vi "Auton Commands.vi"(7 "Roll":dbl, 8 "Turn Angle":dbl, 9 "Distance":dbl=120.0, 10 "Task":u16(ring) items=["Forward", "Backward", "Turn", "Shoot", "Turn Angle", "Roll G", "Roll L"]) -> ()   [LabVIEW 2015]
uses:
  <vilib>/Rock Robotics/Network Tables/NT Read Number.vi
  <vilib>/Rock Robotics/WPI/Utilities/WPI_GetSetVariantRefNum.vi
  <vilib>/addons/control/pid/pid.llb/PID (DBL).vi
  <vilib>/Rock Robotics/Network Tables/NT Write Number.vi
  Robot Global Data.vi
  <vilib>/addons/control/pid/NI_PID_pid.lvlib
  navX Library v2/navX Library v2.lvlib
panel:
  out "Yaw":dbl(graph)
  out "E1 Rate":dbl
  out "E2 Rate":dbl
  in  "Yaw Gains":T1={"proportional gain (Kc)"=0.2, "integral time (Ti, min)"=0.0, "derivative time (Td, min)"=0.0} {"derivative time (Td, min)" format="%.3f"; "integral time (Ti, min)" format="%.3f"; "proportional gain (Kc)" format="%.3f"}
  in  "Speed Gains":T1={"proportional gain (Kc)"=0.65, "integral time (Ti, min)"=0.001, "derivative time (Td, min)"=0.001} {"derivative time (Td, min)" format="%.3f"; "integral time (Ti, min)" format="%.3f"; "proportional gain (Kc)" format="%.3f"}
  in  "Single Turn Gains":T1={"proportional gain (Kc)"=0.12, "integral time (Ti, min)"=0.0, "derivative time (Td, min)"=0.0} {"derivative time (Td, min)" format="%.3f"; "integral time (Ti, min)" format="%.3f"; "proportional gain (Kc)" format="%.3f"}
  out "Right Motor Speed":dbl(graph)
  out "Left Motor Speed":dbl(graph)
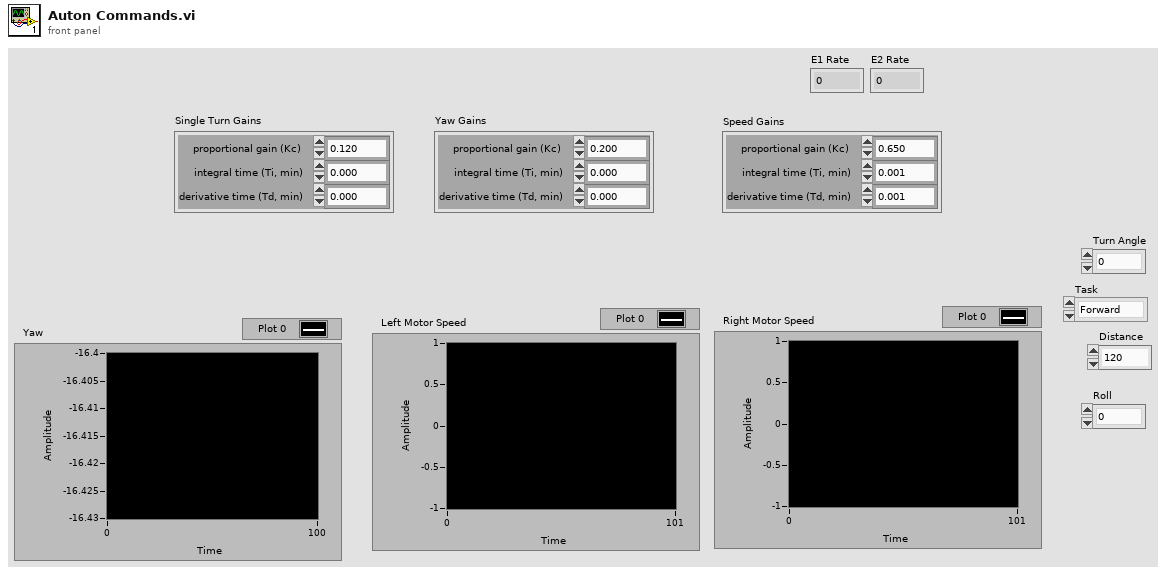
[diagram p1: front panel]
types:
  T1 = cluster{"proportional gain (Kc)":dbl, "integral time (Ti, min)":dbl, "derivative time (Td, min)":dbl}
  T2 = typedef "navX Library v2.lvlib/Z900_navX_DeviceTypeDef.ctl" = cluster{"Interface":cluster{"Protocol":T3, "Update Rate (4Hz-60Hz)":u8, "navX Open TypeDef":variant}, "Notify Packet":refnum<notifier>, "Loop VI Refnum":refnum<vi>, "Ready to Close Occurrence Refnum":refnum<k4>}
  T3 = typedef "navX Library v2.lvlib/Z900_navX_ProtocolTypeDef.ctl" = enum16{"SERIAL", "I2C", "SPI"}
  T4 = typedef "WPI_EncoderDevRef.ctl" = cluster{"DevStatus":errorcluster, "EncoderIndex":T5, "CounterIndex":T6, "DistancePerCount":dbl, "Decoding Type":T7}
  T5 = typedef "FPGA_EncoderIdx.ctl" = enum8{"Enc 0", "Enc 1", "Enc 2", "Enc 3", "Enc 4", "Enc 5", "Enc 6", "Enc 7", "Invalid"}
  T6 = typedef "FPGA_CounterCtrSystemIndex.ctl" = enum8{"Ctr 0", "Ctr 1", "Ctr 2", "Ctr 3", "Ctr 4", "Ctr 5", "Ctr 6", "Ctr 7", "Invalid"}
  T7 = typedef "WPI_EncoderType.ctl" = enum16{"1x", "2x", "4x"}
  T8 = cluster{"Yaw":dbl, "Roll":dbl, "Pitch":dbl, "Heading":dbl, "Fused Heading":dbl}
  T9 = typedef "WPI_RobotDriveDevRef.ctl" = cluster{"DevStatus":errorcluster, "Motors[]":T10[], "Square Inputs":bool, "Max Output":dbl}
  T10 = typedef "WPI_MotorControlDeviceRef.ctl" = cluster{"DeviceStatus":errorcluster, "Type":T11, "PWM":cluster{"PWM Channel":T12, "DeadBand":T13}, "CAN":cluster{"Device Number":u8, "Control Mode":T14, "Semaphore":T15, "Max Vout":dbl, "TalonSRX Control Mode":T16}, "Invert":bool}
  T11 = typedef "WPI_MotorControlType.ctl" = enum16{"PWM", "CAN", "CANTalonSRX"}
  T12 = typedef "FPGA_DIOPWMChannel.ctl" = enum8{"PWM 0", "PWM 1", "PWM 2", "PWM 3", "PWM 4", "PWM 5", "PWM 6", "PWM 7", "PWM 8", "PWM 9", "PWM MXP 0", "PWM MXP 1", "PWM MXP 2", "PWM MXP 3", "PWM MXP 4", "PWM MXP 5", "PWM MXP 6", "PWM MXP 7", "PWM MXP 8", "PWM MXP 9", "Invalid"}
  T13 = typedef "WPI_PWMDeadband.ctl" = cluster{"Name":string, "maxPositivePwm":i32, "minPositivePwm":i32, "centerPwm":i32, "maxNegativePwm":i32, "minNegativePwm":i32, "angularRange":u16}
  T14 = typedef "WPI_CANJaguar_ControlMode.ctl" = enum8{"Percent VBus", "Current", "Speed", "Position", "Voltage"}
  T15 = typedef "Semaphore RefNum" = refnum<k1>
  T16 = typedef "WPI_CANTalonSRX_APIControlMode.ctl" = enum8{"Percent VBus", "Speed", "Position", "Slave", "Unchanged / Invalid", "Voltage Compensation", "Current", "Motion Profile"}
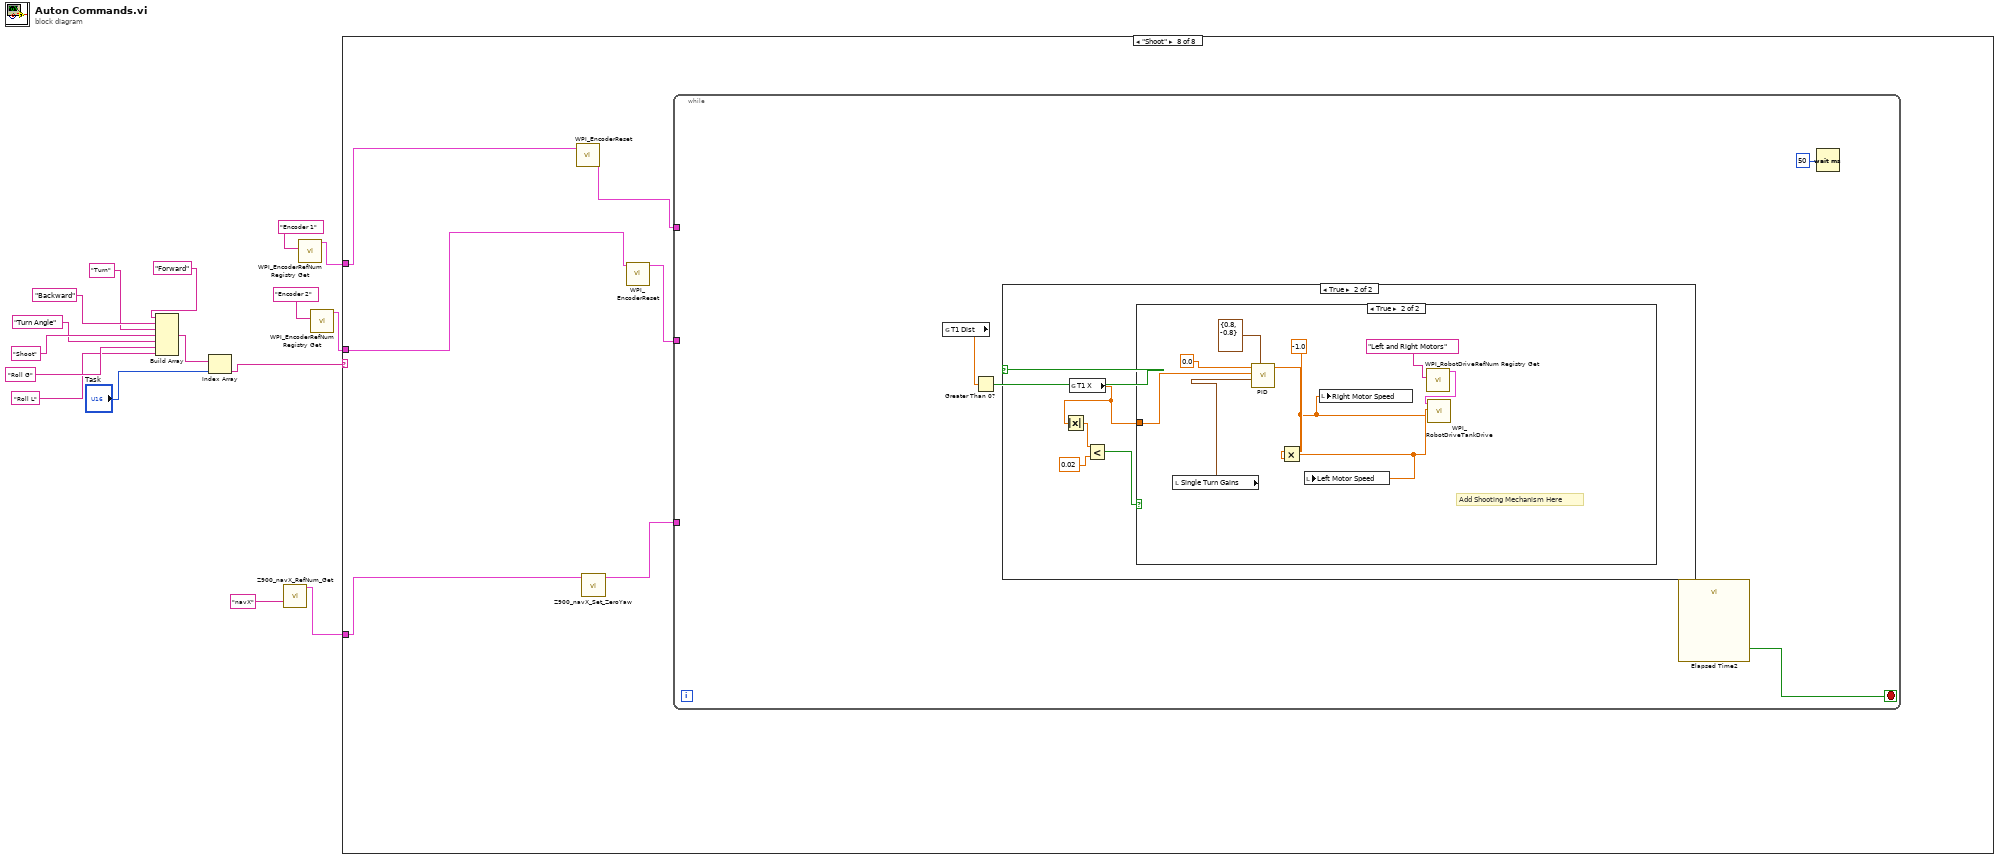
[diagram p0: block diagram]
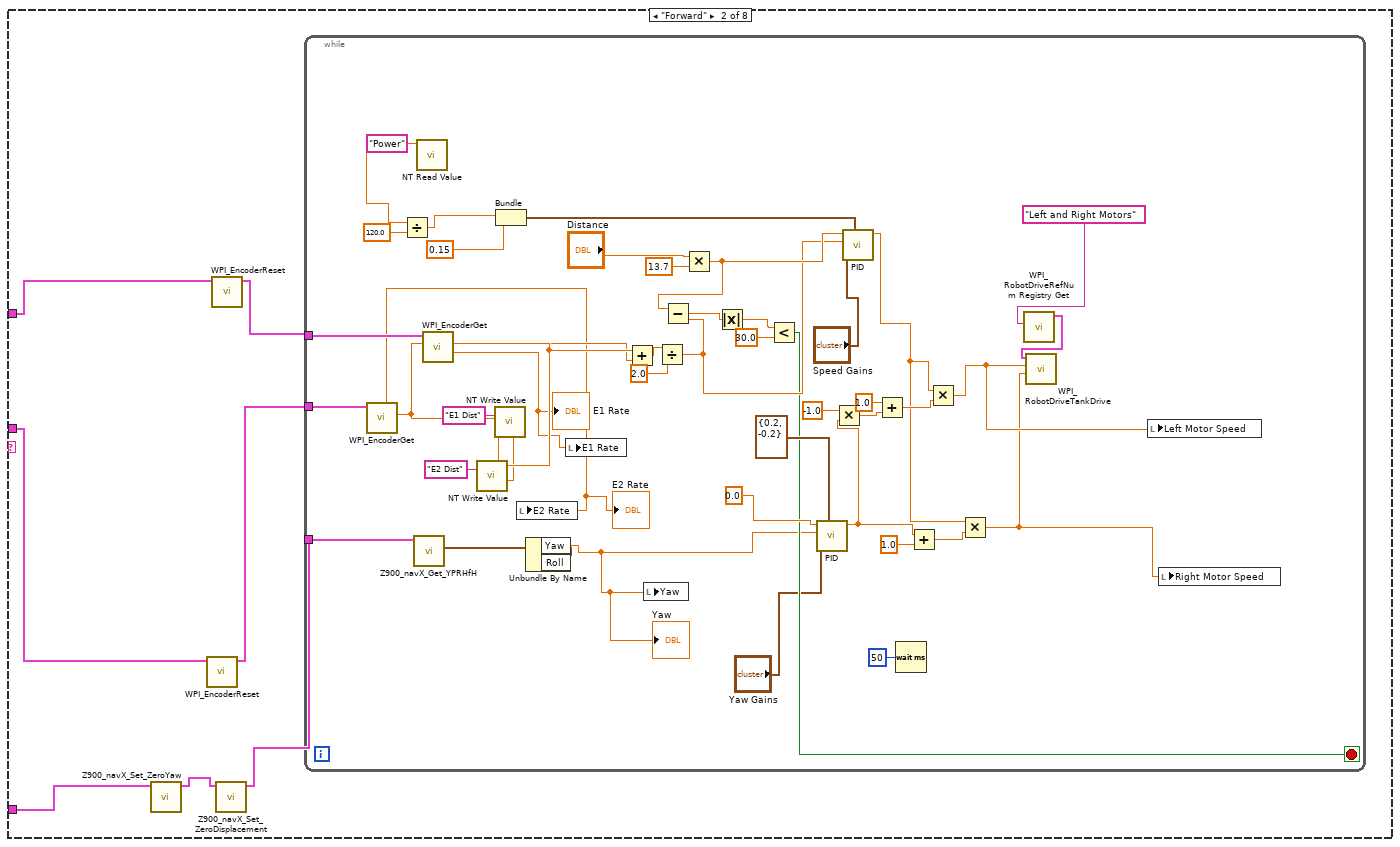
[diagram p3: hidden frame]
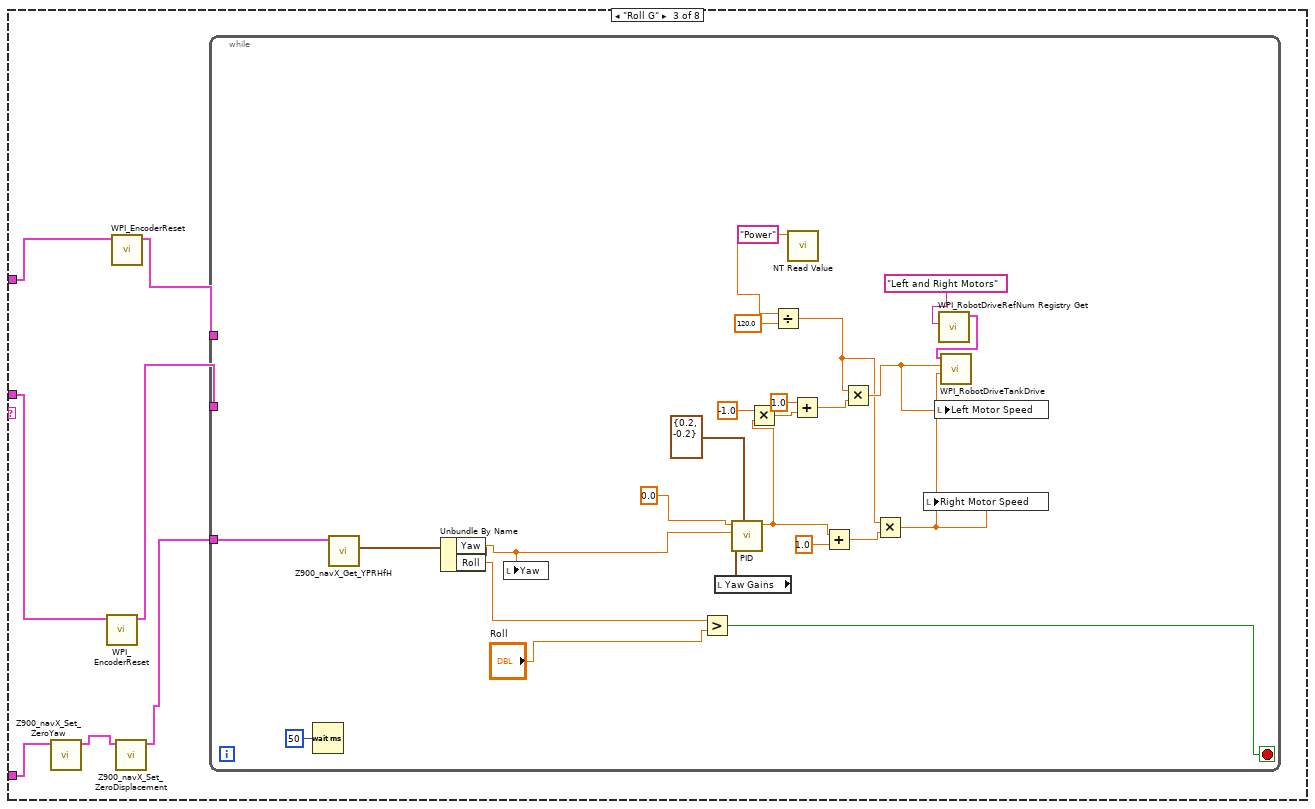
[diagram p4: hidden frame]
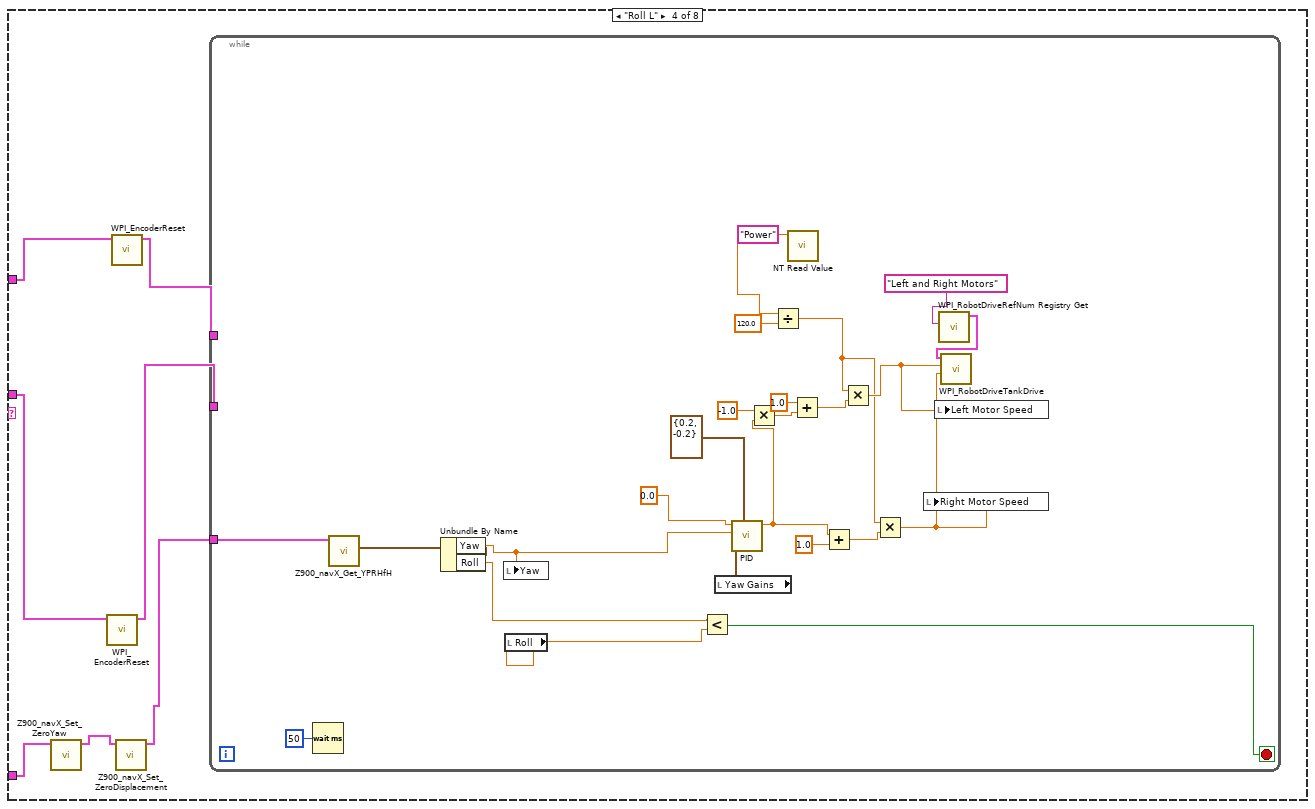
[diagram p5: hidden frame]
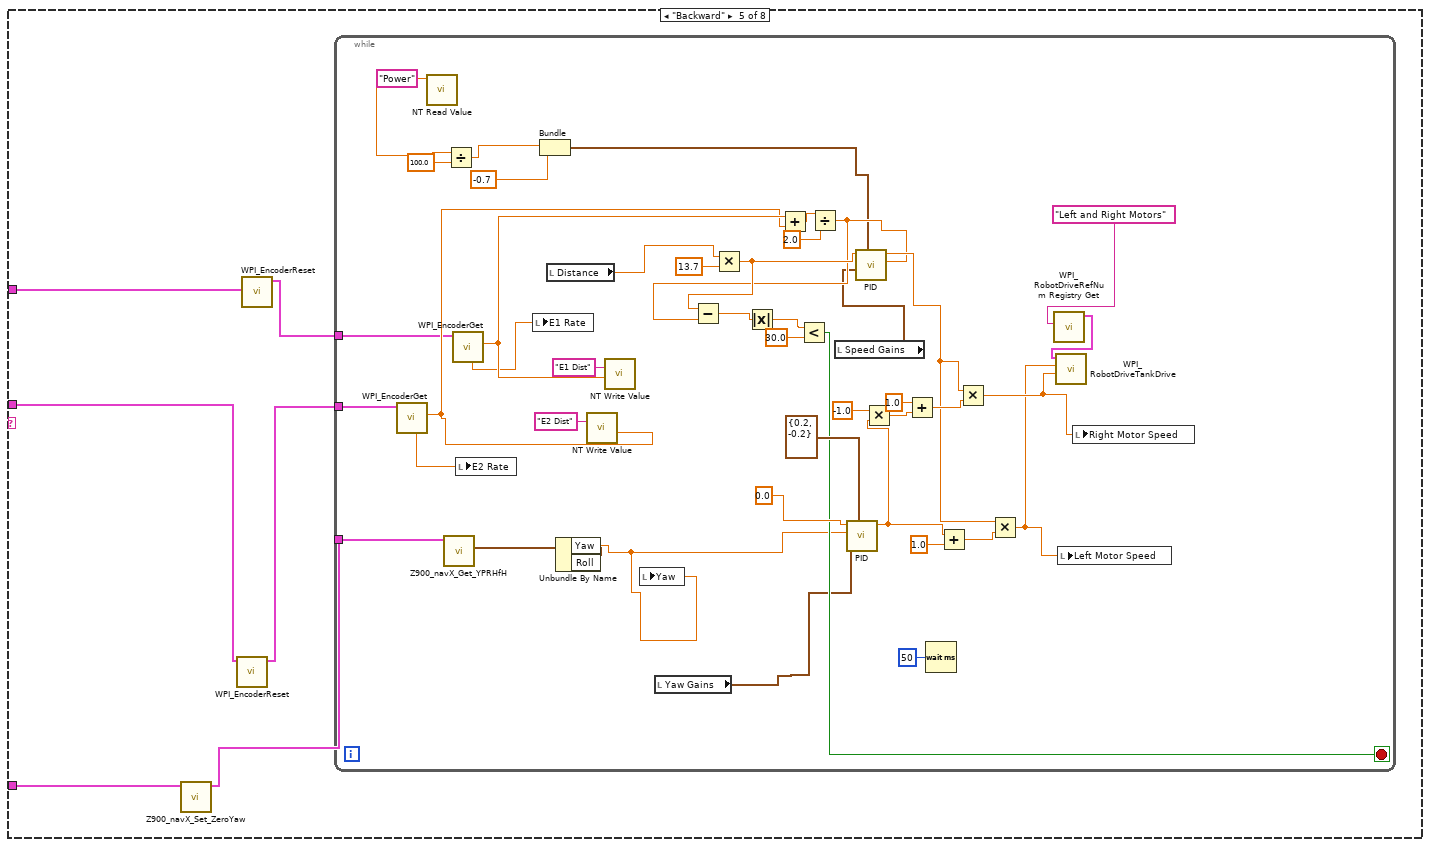
[diagram p6: hidden frame]
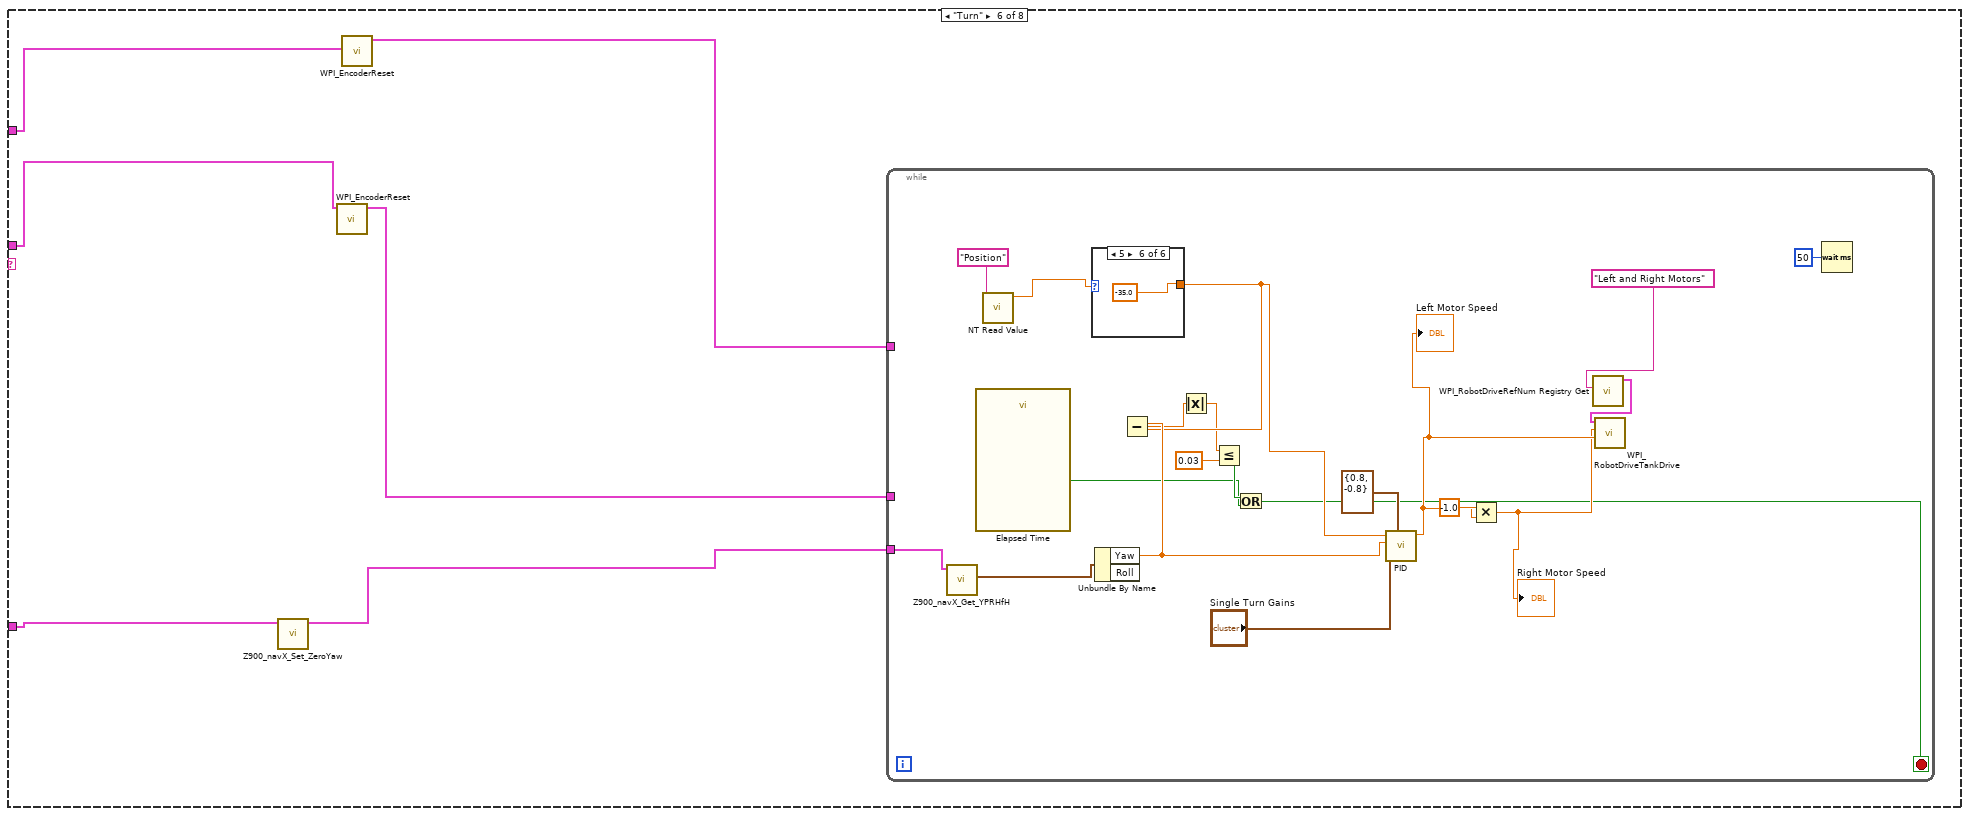
[diagram p7: hidden frame]
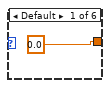
[diagram p8: hidden frame]
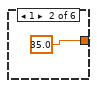
[diagram p9: hidden frame]
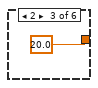
[diagram p10: hidden frame]
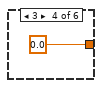
[diagram p11: hidden frame]
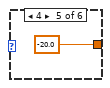
[diagram p12: hidden frame]
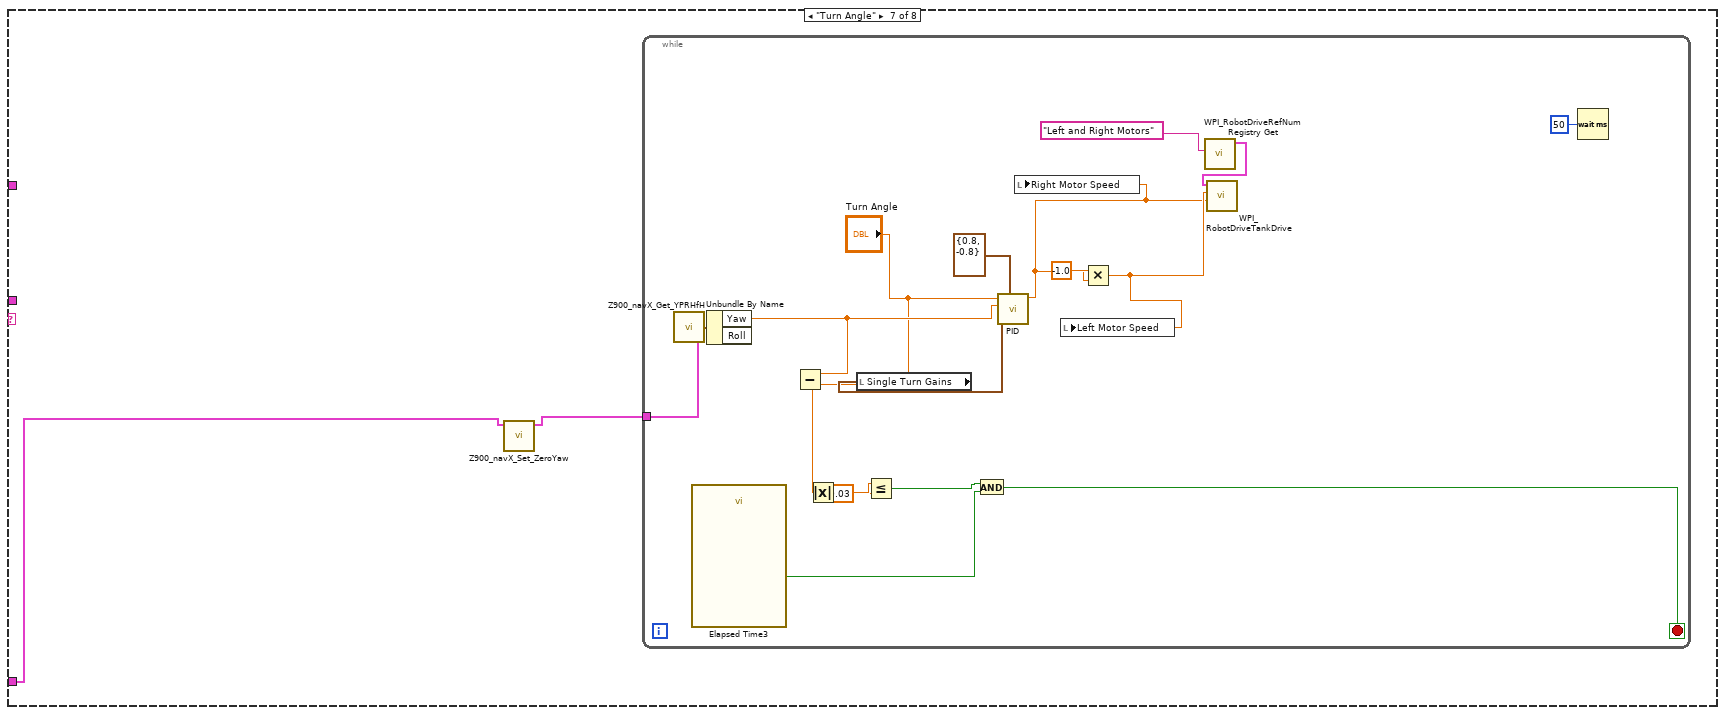
[diagram p13: hidden frame]
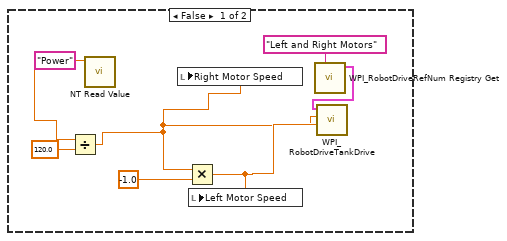
[diagram p14: hidden frame]
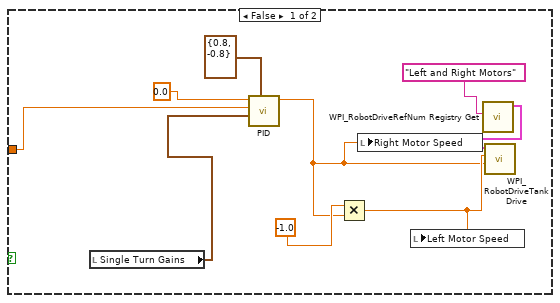
[diagram p15: hidden frame]
diagram:
  n1 = Build Array("Forward", "Backward", "Turn", "Shoot", "Turn Angle" ("element"), "Roll G" ("element"), "Roll L" ("element")) -> (w10:string[])
  n2 = Index Array(array=w10, index="Task") -> (element=w8:string)
  n3 = call "Z900_navX_RefNum_Get.vi"("refnum name"="navX") -> ("navX Device"=w11:T2)  [unwired: 9 in, 1 out]
  n4 = call <vilib>:"WPI_EncoderRefNum Registry Get.vi"("refnum name"="Encoder 1") -> ("EncoderDevRef"=w15:T4)  [unwired: 9 in, 1 out]
  n5 = call <vilib>:"WPI_EncoderRefNum Registry Get.vi"("refnum name"="Encoder 2") -> ("EncoderDevRef"=w13:T4)  [unwired: 9 in, 1 out]
  n6 = case shown="\"Shoot\"" w8 {
    tunnel: w15 -> [_ w21 w73 w105 w134 w184 _ w237]
    tunnel: w13 -> [_ w20 w70 w102 w133 w183 _ w236]
    tunnel: w11 -> [_ w19 w68 w100 w132 w182 w214 w235]
    frame Default {
    }
    frame "Forward" {
      n7 = call "Z900_navX_Set_ZeroYaw.vi"("navX Device"=w19) -> ("navX Device"=w18:T2)  [unwired: 9 in, 1 out]
      n8 = call <vilib>:"WPI_EncoderReset.vi"("EncoderDevRef"=w20) -> ("EncoderDevRef"=w22:T4)  [unwired: 9 in, 1 out]
      n9 = call <vilib>:"WPI_EncoderReset.vi"("EncoderDevRef"=w21) -> ("EncoderDevRef"=w23:T4)  [unwired: 9 in, 1 out]
      n10 = call "Z900_navX_Set_ZeroDisplacement.vi"("navX Device"=w18) -> ("navX Device"=w17:T2)  [unwired: 9 in, 1 out]
      n11 = while {
        tunnel: w23 -> [w34]
        tunnel: w22 -> [w33]
        tunnel: w17 -> [w25]
        stop <- w40 stop-if-true
        n12 = call <vilib>:"WPI_EncoderGet.vi"("EncoderDevRef"=w33) -> ("Distance"=w46:dbl, "Rate"=w32:dbl)  [unwired: 5 in, 4 out]
        "E2 Rate" <- w32
        n13 = call "Z900_navX_Get_YPRHfH.vi"("navX Device"=w25) -> ("YRPHfH"=w62:T8)  [unwired: 7 in, 3 out]
        n14 = call-poly <vilib>:"NT Read Value.vi"("Name"="Power") -> ("Numeric"=w39:dbl)  [unwired: 9 in, 1 out]
        n15 = Divide(x=w39, y=120.0) -> (x/y=w37:dbl)
        n16 = call <vilib>:"WPI_EncoderGet.vi"("EncoderDevRef"=w34) -> ("Distance"=w47:dbl, "Rate"=w31:dbl)  [unwired: 5 in, 4 out]
        "E1 Rate" <- w31
        n17 = call-poly <vilib>:"NT Write Value.vi"("Numeric"=w46, "Name"="E2 Dist") -> ()  [unwired: 9 in, 1 out]
        n18 = call-poly <vilib>:"NT Write Value.vi"("Numeric"=w47, "Name"="E1 Dist") -> ()  [unwired: 9 in, 1 out]
        n19 = Bundle(w37, "output low"=0.15) -> (w35:cluster{dbl, "output low":dbl})  [unwired: 1 in]
        n20 = local write "E2 Rate"(w32) -> ()
        n21 = Unbundle By Name(w62) -> ("Yaw"=w28:dbl)  [unwired: 1 out]
        "Yaw" <- w28
        n22 = local write "E1 Rate"(w31) -> ()
        n23 = Add(x=w47, y=w46) -> (x+y=w61:dbl)
        n24 = local write "Yaw"(w28) -> ()
        n25 = Divide(x=w61, y=2.0) -> (x/y=w44:dbl)
        n26 = Multiply(x="Distance", y=13.7) -> (x*y=w45:dbl)
        n27 = Subtract(x=w45, y=w44) -> (x-y=w43:dbl)
        n28 = Absolute Value(x=w43) -> (abs(x)=w42:dbl)
        n29 = Less?(x=w42, y=30.0) -> (x < y?=w40:bool)
        n30 = call-poly <vilib>:"PID.vi"("output range"=cluster{"output high":dbl, "output low":dbl} {"output high"=0.2, "output low"=-0.2}, "PID gains"="Yaw Gains", "process variable"=w28, "setpoint"=0.0) -> ("output"=w54:dbl)  [unwired: 6 in, 1 out]
        n31 = Multiply(x=-1.0, y=w54) -> (x*y=w55:dbl)
        n32 = call-poly <vilib>:"PID.vi"("output range"=w35, "PID gains"="Speed Gains", "process variable"=w44, "setpoint"=w45) -> ("output"=w51:dbl)  [unwired: 6 in, 1 out]
        n33 = Add(x=1.0, y=w55) -> (x+y=w56:dbl)
        n34 = Wait (ms)(milliseconds to wait=u32 50) -> ()  [unwired: 1 out]
        n35 = Add(x=w54, y=1.0) -> (x+y=w57:dbl)
        n36 = Multiply(x=w51, y=w56) -> (x*y=w49:dbl)
        n37 = Multiply(x=w51, y=w57) -> (x*y=w24:dbl)
        n38 = call <vilib>:"WPI_RobotDriveRefNum Registry Get.vi"("refnum name"="Left and Right Motors") -> ("RobotDriveDevRef"=w64:T9)  [unwired: 9 in, 1 out]
        n39 = call <vilib>:"WPI_RobotDriveTankDrive.vi"("Right axis value"=w24, "Left axis value"=w49, "RobotDriveDevRef"=w64) -> ()  [unwired: 6 in, 3 out]
        n40 = local write "Left Motor Speed"(w49) -> ()
        n41 = local write "Right Motor Speed"(w24) -> ()
      }
    }
    frame "Roll G" {
      n42 = call "Z900_navX_Set_ZeroYaw.vi"("navX Device"=w68) -> ("navX Device"=w74:T2)  [unwired: 9 in, 1 out]
      n43 = call <vilib>:"WPI_EncoderReset.vi"("EncoderDevRef"=w70) -> ("EncoderDevRef"=w71:T4)  [unwired: 9 in, 1 out]
      n44 = call <vilib>:"WPI_EncoderReset.vi"("EncoderDevRef"=w73) -> ("EncoderDevRef"=w72:T4)  [unwired: 9 in, 1 out]
      n45 = call "Z900_navX_Set_ZeroDisplacement.vi"("navX Device"=w74) -> ("navX Device"=w69:T2)  [unwired: 9 in, 1 out]
      n46 = while {
        tunnel: w72 -> [_]
        tunnel: w71 -> [_]
        tunnel: w69 -> [w82]
        stop <- w76 stop-if-true
        n47 = Wait (ms)(milliseconds to wait=u32 50) -> ()  [unwired: 1 out]
        n48 = call "Z900_navX_Get_YPRHfH.vi"("navX Device"=w82) -> ("YRPHfH"=w96:T8)  [unwired: 7 in, 3 out]
        n49 = Unbundle By Name(w96) -> ("Yaw"=w80:dbl, "Roll"=w77:dbl)
        n50 = local write "Yaw"(w80) -> ()
        n51 = Greater?(x=w77, y="Roll") -> (0:w76:bool)
        n52 = local read "Yaw Gains"() -> (w81:T1)
        n53 = call-poly <vilib>:"PID.vi"("output range"=cluster{"output high":dbl, "output low":dbl} {"output high"=0.2, "output low"=-0.2}, "PID gains"=w81, "process variable"=w80, "setpoint"=0.0) -> ("output"=w90:dbl)  [unwired: 6 in, 1 out]
        n54 = Multiply(x=-1.0, y=w90) -> (x*y=w91:dbl)
        n55 = call-poly <vilib>:"NT Read Value.vi"("Name"="Power") -> ("Numeric"=w85:dbl)  [unwired: 9 in, 1 out]
        n56 = Divide(x=w85, y=120.0) -> (x/y=w79:dbl)
        n57 = Add(x=1.0, y=w91) -> (x+y=w92:dbl)
        n58 = Add(x=w90, y=1.0) -> (x+y=w93:dbl)
        n59 = Multiply(x=w79, y=w92) -> (x*y=w87:dbl)
        n60 = Multiply(x=w79, y=w93) -> (x*y=w78:dbl)
        n61 = local write "Right Motor Speed"(w78) -> ()
        n62 = local write "Left Motor Speed"(w87) -> ()
        n63 = call <vilib>:"WPI_RobotDriveRefNum Registry Get.vi"("refnum name"="Left and Right Motors") -> ("RobotDriveDevRef"=w98:T9)  [unwired: 9 in, 1 out]
        n64 = call <vilib>:"WPI_RobotDriveTankDrive.vi"("Right axis value"=w78, "Left axis value"=w87, "RobotDriveDevRef"=w98) -> ()  [unwired: 6 in, 3 out]
      }
    }
    frame "Roll L" {
      n65 = call "Z900_navX_Set_ZeroYaw.vi"("navX Device"=w100) -> ("navX Device"=w106:T2)  [unwired: 9 in, 1 out]
      n66 = call <vilib>:"WPI_EncoderReset.vi"("EncoderDevRef"=w102) -> ("EncoderDevRef"=w103:T4)  [unwired: 9 in, 1 out]
      n67 = call <vilib>:"WPI_EncoderReset.vi"("EncoderDevRef"=w105) -> ("EncoderDevRef"=w104:T4)  [unwired: 9 in, 1 out]
      n68 = call "Z900_navX_Set_ZeroDisplacement.vi"("navX Device"=w106) -> ("navX Device"=w101:T2)  [unwired: 9 in, 1 out]
      n69 = while {
        tunnel: w104 -> [_]
        tunnel: w103 -> [_]
        tunnel: w101 -> [w114]
        stop <- w108 stop-if-true
        n70 = Wait (ms)(milliseconds to wait=u32 50) -> ()  [unwired: 1 out]
        n71 = call "Z900_navX_Get_YPRHfH.vi"("navX Device"=w114) -> ("YRPHfH"=w128:T8)  [unwired: 7 in, 3 out]
        n72 = Unbundle By Name(w128) -> ("Yaw"=w112:dbl, "Roll"=w109:dbl)
        n73 = local write "Yaw"(w112) -> ()
        n74 = local read "Roll"() -> (w107:dbl)
        n75 = Less?(x=w109, y=w107) -> (x < y?=w108:bool)
        n76 = local read "Yaw Gains"() -> (w113:T1)
        n77 = call-poly <vilib>:"PID.vi"("output range"=cluster{"output high":dbl, "output low":dbl} {"output high"=0.2, "output low"=-0.2}, "PID gains"=w113, "process variable"=w112, "setpoint"=0.0) -> ("output"=w122:dbl)  [unwired: 6 in, 1 out]
        n78 = Multiply(x=-1.0, y=w122) -> (x*y=w123:dbl)
        n79 = call-poly <vilib>:"NT Read Value.vi"("Name"="Power") -> ("Numeric"=w117:dbl)  [unwired: 9 in, 1 out]
        n80 = Divide(x=w117, y=120.0) -> (x/y=w111:dbl)
        n81 = Add(x=1.0, y=w123) -> (x+y=w124:dbl)
        n82 = Add(x=w122, y=1.0) -> (x+y=w125:dbl)
        n83 = Multiply(x=w111, y=w124) -> (x*y=w119:dbl)
        n84 = Multiply(x=w111, y=w125) -> (x*y=w110:dbl)
        n85 = local write "Right Motor Speed"(w110) -> ()
        n86 = local write "Left Motor Speed"(w119) -> ()
        n87 = call <vilib>:"WPI_RobotDriveRefNum Registry Get.vi"("refnum name"="Left and Right Motors") -> ("RobotDriveDevRef"=w130:T9)  [unwired: 9 in, 1 out]
        n88 = call <vilib>:"WPI_RobotDriveTankDrive.vi"("Right axis value"=w110, "Left axis value"=w119, "RobotDriveDevRef"=w130) -> ()  [unwired: 6 in, 3 out]
      }
    }
    frame "Backward" {
      n89 = call "Z900_navX_Set_ZeroYaw.vi"("navX Device"=w132) -> ("navX Device"=w135:T2)  [unwired: 9 in, 1 out]
      n90 = call <vilib>:"WPI_EncoderReset.vi"("EncoderDevRef"=w133) -> ("EncoderDevRef"=w136:T4)  [unwired: 9 in, 1 out]
      n91 = call <vilib>:"WPI_EncoderReset.vi"("EncoderDevRef"=w134) -> ("EncoderDevRef"=w137:T4)  [unwired: 9 in, 1 out]
      n92 = while {
        tunnel: w137 -> [w149]
        tunnel: w136 -> [w148]
        tunnel: w135 -> [w147]
        stop <- w155 stop-if-true
        n93 = call <vilib>:"WPI_EncoderGet.vi"("EncoderDevRef"=w148) -> ("Distance"=w161:dbl, "Rate"=w143:dbl)  [unwired: 5 in, 4 out]
        n94 = call-poly <vilib>:"NT Read Value.vi"("Name"="Power") -> ("Numeric"=w154:dbl)  [unwired: 9 in, 1 out]
        n95 = call "Z900_navX_Get_YPRHfH.vi"("navX Device"=w147) -> ("YRPHfH"=w176:T8)  [unwired: 7 in, 3 out]
        n96 = Divide(x=w154, y=100.0) -> (x/y=w152:dbl)
        n97 = call <vilib>:"WPI_EncoderGet.vi"("EncoderDevRef"=w149) -> ("Distance"=w162:dbl, "Rate"=w142:dbl)  [unwired: 5 in, 4 out]
        n98 = local write "E2 Rate"(w143) -> ()
        n99 = local write "E1 Rate"(w142) -> ()
        n100 = Bundle(w152, "output low"=-0.7) -> (w150:cluster{dbl, "output low":dbl})  [unwired: 1 in]
        n101 = local read "Distance"() -> (w141:dbl)
        n102 = Unbundle By Name(w176) -> ("Yaw"=w145:dbl)  [unwired: 1 out]
        n103 = call-poly <vilib>:"NT Write Value.vi"("Numeric"=w161, "Name"="E2 Dist") -> ()  [unwired: 9 in, 1 out]
        n104 = call-poly <vilib>:"NT Write Value.vi"("Numeric"=w162, "Name"="E1 Dist") -> ()  [unwired: 9 in, 1 out]
        n105 = local write "Yaw"(w145) -> ()
        n106 = local read "Yaw Gains"() -> (w144:T1)
        n107 = Multiply(x=w141, y=13.7) -> (x*y=w160:dbl)
        n108 = Add(x=w162, y=w161) -> (x+y=w175:dbl)
        n109 = Divide(x=w175, y=2.0) -> (x/y=w159:dbl)
        n110 = Subtract(x=w160, y=w159) -> (x-y=w158:dbl)
        n111 = Absolute Value(x=w158) -> (abs(x)=w157:dbl)
        n112 = Less?(x=w157, y=30.0) -> (x < y?=w155:bool)
        n113 = local read "Speed Gains"() -> (w138:T1)
        n114 = call-poly <vilib>:"PID.vi"("output range"=cluster{"output high":dbl, "output low":dbl} {"output high"=0.2, "output low"=-0.2}, "PID gains"=w144, "process variable"=w145, "setpoint"=0.0) -> ("output"=w168:dbl)  [unwired: 6 in, 1 out]
        n115 = call-poly <vilib>:"PID.vi"("output range"=w150, "PID gains"=w138, "process variable"=w159, "setpoint"=w160) -> ("output"=w165:dbl)  [unwired: 6 in, 1 out]
        n116 = Multiply(x=-1.0, y=w168) -> (x*y=w169:dbl)
        n117 = Add(x=1.0, y=w169) -> (x+y=w170:dbl)
        n118 = Wait (ms)(milliseconds to wait=u32 50) -> ()  [unwired: 1 out]
        n119 = Add(x=w168, y=1.0) -> (x+y=w171:dbl)
        n120 = Multiply(x=w165, y=w170) -> (x*y=w140:dbl)
        n121 = Multiply(x=w165, y=w171) -> (x*y=w139:dbl)
        n122 = call <vilib>:"WPI_RobotDriveRefNum Registry Get.vi"("refnum name"="Left and Right Motors") -> ("RobotDriveDevRef"=w178:T9)  [unwired: 9 in, 1 out]
        n123 = call <vilib>:"WPI_RobotDriveTankDrive.vi"("Right axis value"=w140, "Left axis value"=w139, "RobotDriveDevRef"=w178) -> ()  [unwired: 6 in, 3 out]
        n124 = local write "Left Motor Speed"(w139) -> ()
        n125 = local write "Right Motor Speed"(w140) -> ()
      }
    }
    frame "Turn" {
      n126 = call "Z900_navX_Set_ZeroYaw.vi"("navX Device"=w182) -> ("navX Device"=w185:T2)  [unwired: 9 in, 1 out]
      n127 = call <vilib>:"WPI_EncoderReset.vi"("EncoderDevRef"=w183) -> ("EncoderDevRef"=w186:T4)  [unwired: 9 in, 1 out]
      n128 = call <vilib>:"WPI_EncoderReset.vi"("EncoderDevRef"=w184) -> ("EncoderDevRef"=w187:T4)  [unwired: 9 in, 1 out]
      n129 = while {
        tunnel: w187 -> [_]
        tunnel: w186 -> [_]
        tunnel: w185 -> [w203]
        stop <- w188 stop-if-true
        n130 = call "Z900_navX_Get_YPRHfH.vi"("navX Device"=w203) -> ("YRPHfH"=w202:T8)  [unwired: 7 in, 3 out]
        n131 = call "Elapsed Time"() -> ("Time has Elapsed"=w189:bool)  [unwired: 12 in, 7 out]
        n132 = call-poly <vilib>:"NT Read Value.vi"("Name"="Position") -> ("Numeric"=w199:dbl)  [unwired: 9 in, 1 out]
        n133 = case shown="5" w199 {
          tunnel: [0.0 35.0 20.0 0.0 -20.0 -35.0] -> w194
          frame Default {
          }
          frame 1 {
          }
          frame 2 {
          }
          frame 3 {
          }
          frame 4 {
          }
          frame 5 {
          }
        }
        n134 = Unbundle By Name(w202) -> ("Yaw"=w195:dbl)  [unwired: 1 out]
        n135 = Subtract(x=w195, y=w194) -> (x-y=w193:dbl)
        n136 = Absolute Value(x=w193) -> (abs(x)=w192:dbl)
        n137 = Less Or Equal?(x=w192, y=0.03) -> (x <= y?=w190:bool)
        n138 = Or(x=w190, y=w189) -> (x .or. y?=w188:bool)
        n139 = call-poly <vilib>:"PID.vi"("output range"=cluster{"output high":dbl, "output low":dbl} {"output high"=0.8, "output low"=-0.8}, "PID gains"="Single Turn Gains", "process variable"=w195, "setpoint"=w194) -> ("output"=w197:dbl)  [unwired: 6 in, 1 out]
        "Left Motor Speed" <- w197
        n140 = Multiply(x=-1.0, y=w197) -> (x*y=w196:dbl)
        "Right Motor Speed" <- w196
        n141 = call <vilib>:"WPI_RobotDriveRefNum Registry Get.vi"("refnum name"="Left and Right Motors") -> ("RobotDriveDevRef"=w206:T9)  [unwired: 9 in, 1 out]
        n142 = call <vilib>:"WPI_RobotDriveTankDrive.vi"("Right axis value"=w197, "Left axis value"=w196, "RobotDriveDevRef"=w206) -> ()  [unwired: 6 in, 3 out]
        n143 = Wait (ms)(milliseconds to wait=u32 50) -> ()  [unwired: 1 out]
      }
    }
    frame "Turn Angle" {
      n144 = call "Z900_navX_Set_ZeroYaw.vi"("navX Device"=w214) -> ("navX Device"=w215:T2)  [unwired: 9 in, 1 out]
      n145 = while {
        tunnel: w215 -> [w229]
        stop <- w216 stop-if-true
        n146 = call "Z900_navX_Get_YPRHfH.vi"("navX Device"=w229) -> ("YRPHfH"=w228:T8)  [unwired: 7 in, 3 out]
        n147 = call "Elapsed Time3"() -> ("Time has Elapsed"=w217:bool)  [unwired: 12 in, 7 out]
        n148 = Unbundle By Name(w228) -> ("Yaw"=w223:dbl)  [unwired: 1 out]
        n149 = Subtract(x=w223, y="Turn Angle") -> (x-y=w221:dbl)
        n150 = Absolute Value(x=w221) -> (abs(x)=w220:dbl)
        n151 = local read "Single Turn Gains"() -> (w226:T1)
        n152 = Less Or Equal?(x=w220, y=0.03) -> (x <= y?=w218:bool)
        n153 = And(x=w218, y=w217) -> (x .and. y?=w216:bool)
        n154 = call-poly <vilib>:"PID.vi"("output range"=cluster{"output high":dbl, "output low":dbl} {"output high"=0.8, "output low"=-0.8}, "PID gains"=w226, "process variable"=w223, "setpoint"="Turn Angle") -> ("output"=w224:dbl)  [unwired: 6 in, 1 out]
        n155 = local write "Right Motor Speed"(w224) -> ()
        n156 = Multiply(x=-1.0, y=w224) -> (x*y=w225:dbl)
        n157 = local write "Left Motor Speed"(w225) -> ()
        n158 = call <vilib>:"WPI_RobotDriveRefNum Registry Get.vi"("refnum name"="Left and Right Motors") -> ("RobotDriveDevRef"=w232:T9)  [unwired: 9 in, 1 out]
        n159 = call <vilib>:"WPI_RobotDriveTankDrive.vi"("Right axis value"=w224, "Left axis value"=w225, "RobotDriveDevRef"=w232) -> ()  [unwired: 6 in, 3 out]
        n160 = Wait (ms)(milliseconds to wait=u32 50) -> ()  [unwired: 1 out]
      }
    }
    frame "Shoot" {
      n161 = call <vilib>:"WPI_EncoderReset.vi"("EncoderDevRef"=w237) -> ("EncoderDevRef"=w234:T4)  [unwired: 9 in, 1 out]
      n162 = call "Z900_navX_Set_ZeroYaw.vi"("navX Device"=w235) -> ("navX Device"=w238:T2)  [unwired: 9 in, 1 out]
      n163 = call <vilib>:"WPI_EncoderReset.vi"("EncoderDevRef"=w236) -> ("EncoderDevRef"=w239:T4)  [unwired: 9 in, 1 out]
      n164 = while {
        tunnel: w234 -> [_]
        tunnel: w239 -> [_]
        tunnel: w238 -> [_]
        stop <- w242 stop-if-true
        n165 = global read "Robot Global Data.vi" "T1 Dist"() -> (w241:dbl)
        n166 = Greater Than 0?(x=w241) -> (x > 0?=w240:bool)
        n167 = case shown="True" w240 {
          frame False {
            n168 = call-poly <vilib>:"NT Read Value.vi"("Name"="Power") -> ("Numeric"=w248:dbl)  [unwired: 9 in, 1 out]
            n169 = Divide(x=w248, y=120.0) -> (x/y=w244:dbl)
            n170 = local write "Right Motor Speed"(w244) -> ()
            n171 = Multiply(x=w244, y=-1.0) -> (x*y=w245:dbl)
            n172 = local write "Left Motor Speed"(w245) -> ()
            n173 = call <vilib>:"WPI_RobotDriveRefNum Registry Get.vi"("refnum name"="Left and Right Motors") -> ("RobotDriveDevRef"=w250:T9)  [unwired: 9 in, 1 out]
            n174 = call <vilib>:"WPI_RobotDriveTankDrive.vi"("Right axis value"=w245, "Left axis value"=w244, "RobotDriveDevRef"=w250) -> ()  [unwired: 6 in, 3 out]
          }
          frame True {
            n175 = global read "Robot Global Data.vi" "T1 X"() -> (w255:dbl)
            n176 = Absolute Value(x=w255) -> (abs(x)=w254:dbl)
            n177 = Less?(x=w254, y=0.02) -> (x < y?=w252:bool)
            n178 = case shown="True" w252 {
              tunnel: w255 -> [w259 w268]
              frame False {
                n179 = local read "Single Turn Gains"() -> (w258:T1)
                n180 = call-poly <vilib>:"PID.vi"("output range"=cluster{"output high":dbl, "output low":dbl} {"output high"=0.8, "output low"=-0.8}, "PID gains"=w258, "process variable"=w259, "setpoint"=0.0) -> ("output"=w256:dbl)  [unwired: 6 in, 1 out]
                n181 = Multiply(x=-1.0, y=w256) -> (x*y=w257:dbl)
                n182 = local write "Right Motor Speed"(w256) -> ()
                n183 = local write "Left Motor Speed"(w257) -> ()
                n184 = call <vilib>:"WPI_RobotDriveRefNum Registry Get.vi"("refnum name"="Left and Right Motors") -> ("RobotDriveDevRef"=w262:T9)  [unwired: 9 in, 1 out]
                n185 = call <vilib>:"WPI_RobotDriveTankDrive.vi"("Right axis value"=w256, "Left axis value"=w257, "RobotDriveDevRef"=w262) -> ()  [unwired: 6 in, 3 out]
              }
              frame True {
                # "Add Shooting Mechanism Here"
                n186 = local read "Single Turn Gains"() -> (w267:T1)
                n187 = call-poly <vilib>:"PID.vi"("output range"=cluster{"output high":dbl, "output low":dbl} {"output high"=0.8, "output low"=-0.8}, "PID gains"=w267, "process variable"=w268, "setpoint"=0.0) -> ("output"=w265:dbl)  [unwired: 6 in, 1 out]
                n188 = Multiply(x=-1.0, y=w265) -> (x*y=w266:dbl)
                n189 = local write "Left Motor Speed"(w266) -> ()
                n190 = local write "Right Motor Speed"(w265) -> ()
                n191 = call <vilib>:"WPI_RobotDriveRefNum Registry Get.vi"("refnum name"="Left and Right Motors") -> ("RobotDriveDevRef"=w271:T9)  [unwired: 9 in, 1 out]
                n192 = call <vilib>:"WPI_RobotDriveTankDrive.vi"("Right axis value"=w265, "Left axis value"=w266, "RobotDriveDevRef"=w271) -> ()  [unwired: 6 in, 3 out]
              }
            }
          }
        }
        n193 = call "Elapsed Time2"() -> ("Time has Elapsed"=w242:bool)  [unwired: 12 in, 7 out]
        n194 = Wait (ms)(milliseconds to wait=u32 50) -> ()  [unwired: 1 out]
      }
    }
  }
